vi "Gaussian Window (DBL).vi"(10 "standard deviation":dbl=0.2, 11 "X":dbl[](array[numeric])) -> (0 "error":i32, 3 "Windowed X":dbl[](array[numeric]))   [LabVIEW 2020, in "NI_AALPro.lvlib"]
doc: "Applies an asymmetrical Gaussian window to the input sequence <B>X</B>. Wire data to the <B>X</B> input to determine the polymorphic instance to use or manually select the instance."
uses:
  NI_AALPro.lvlib
  <resource>/lvanlys.dll
panel:
  # "Gaussian Window"
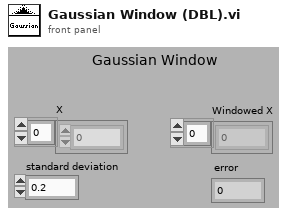
[diagram p1: front panel]
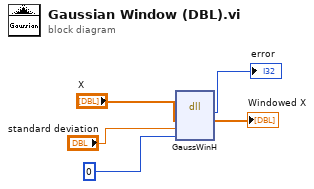
[diagram p0: block diagram]
diagram:
  n1 = dll-call lib="C:/Program Files (x86)/National Instruments/LabVIEW 2020/resource/lvanlys.*" fn="GaussWinH"("X"="X", "stdDev"="standard deviation", "symmetric"=0) -> (→"error":i32, "X"=→"Windowed X":dbl[])  [unwired: 5 in, 2 out]
